vi "MiniProject.vi"() -> ()   [LabVIEW 2021]
panel:
  out "LDR Estimated Lux":dbl
  out "Calculated (V)":dbl
  out "Too Dim 2":bool
  out "Too Bright 2":bool
  out "Raw Voltage (V)":dbl
  out "Average Measured (V)":dbl
  out "Too Dim":bool
  out "Too Bright":bool
  in  "Offset (%)":dbl min=0.0 max=1.0 step=0.01
  out "Reading Range":T1(graph)
  out "LDR Measured Resistance (kOhms)":dbl
  out "Conditioned Signal":T1(graph)
  in  "Stop":bool
  out "Highest Measured Value (V)":dbl
  out "Lowest Measured Value (V)":dbl
  # "500 lux (4.55V)"
  # "100 lux (3.33V)"
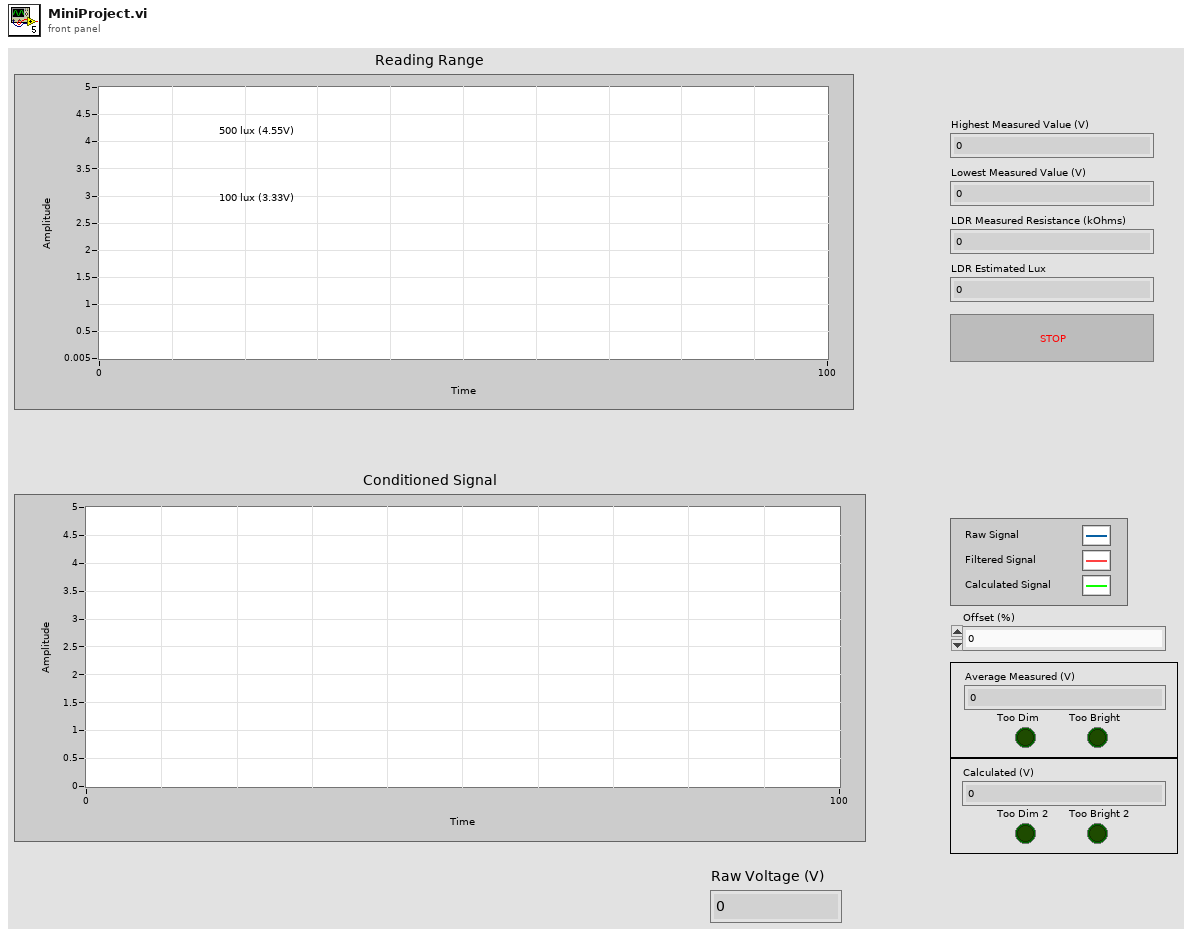
[diagram p1: front panel]
types:
  T1 = cluster{"Voltage Output 1":dbl, "Voltage Output 2":dbl, "Calculated":dbl}
  T2 = enum16{"open", "replace", "create", "open or create", "replace or create", "replace or create with confirmation"}
  T3 = cluster{"Voltage Output 2":dbl, "Min Value":dbl, "Max Value":dbl}
  T4 = cluster{"Voltage Output 2":dbl, dbl, "Calculated":dbl}
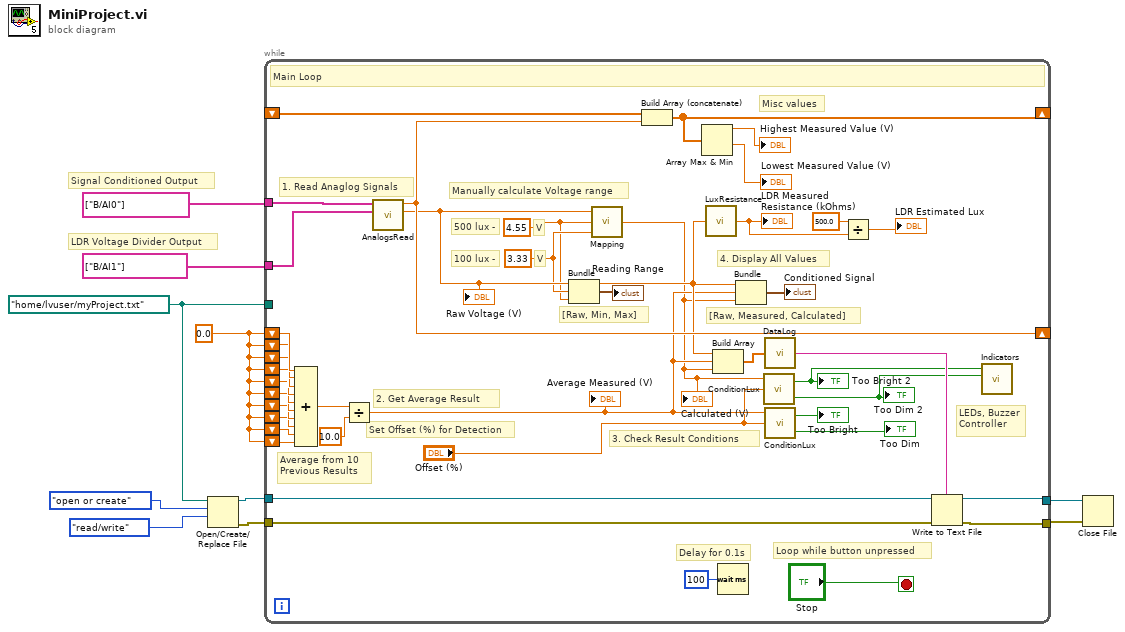
[diagram p0: block diagram]
diagram:
  w5 = path "/home/lvuser/myProject.txt" ("Logfile Location Path")
  w8 = 0.0 ("Voltage Output 2")
  # "LDR Voltage Divider Output"
  # "Signal Conditioned Output"
  n1 = Open/Create/Replace File(file path (use dialog)=w5, operation (0:open)=T2."open or create", access (0:read/write)=enum16{"read/write", "read-only", "write-only"}."read/write") -> (refnum out=w2:refnum<file>, error out=w1:errorcluster)  [unwired: 3 in, 1 out]
  n2 = while {
    tunnel: tag[] ["B/AI0"] ("Analog Input 1") -> [w34]
    tunnel: tag[] ["B/AI1"] ("Analog Input 2") -> [w33]
    shift-right: [w32] -> _
    shift-left: w8 -> [w52]
    shift-left: w8 -> [w51]
    shift-left: w8 -> [w50]
    shift-left: w8 -> [w49]
    shift-left: w8 -> [w48]
    shift-left: w8 -> [w47]
    shift-left: w8 -> [w46]
    shift-left: w8 -> [w45]
    shift-left: w8 -> [w44]
    shift-left: w8 -> [w43]
    shift-right: [w37] -> _
    shift-left: _ -> [w38]
    tunnel: w5 -> [_]
    tunnel: [w17] -> w7
    tunnel: [w16] -> w6
    tunnel: w2 -> [w14]
    tunnel: w1 -> [w13]
    stop <- "Stop" stop-if-true
    w28 = 3.33 ("Min Value")
    w27 = 4.55 ("Max Value")
    # "LEDs, Buzzer\nController"
    # "Set Offset (%) for Detection"
    # "4. Display All Values"
    # "3. Check Result Conditions"
    # "Delay for 0.1s"
    # "2. Get Average Result"
    # "Loop while button unpressed"
    # "V"
    # "V"
    # "1. Read Anaglog Signals"
    # "Misc values"
    # "[Raw, Measured, Calculated]"
    # "[Raw, Min, Max]"
    # "100 lux -"
    # "500 lux -"
    # "Manually calculate Voltage range"
    # "Average from 10 \nPrevious Results"
    # "Main Loop"
    n3 = Compound Arithmetic op=ADD(w52, w51, w50, w49, w48, w47, w46, w45, w44, w43) -> (w42:dbl)
    n4 = Divide(x=w42, y=10.0) -> (x/y=w26:dbl)
    "Average Measured (V)" <- w26
    n5 = call "AnalogsRead.vi"("Analog Input 2"=w33, "Analog Input 1"=w34) -> ("Voltage Output 2"=w30:dbl, "Voltage Output 1"=w32:dbl)  [unwired: 7 in, 1 out]
    "Raw Voltage (V)" <- w30
    n6 = Bundle("Voltage Output 2"=w30, "Min Value"=w28, "Max Value"=w27) -> (→"Reading Range":T3)  [unwired: 1 in]
    n7 = call "Mapping.vi"("Min Value"=w28, "Max Value"=w27, "Raw Signal"=w30) -> ("Calculated"=w22:dbl)
    "Calculated (V)" <- w22
    n8 = Build Array (concatenate)(w38, w32) -> (w37:dbl[])
    n9 = Array Max & Min(array=w37) -> (max value=→"Highest Measured Value (V)":dbl, min value=→"Lowest Measured Value (V)":dbl)  [unwired: 2 out]
    n10 = call "LuxResistance.vi"("Vout"=w30) -> ("Resistance (kOhms)"=w21:dbl)
    "LDR Measured Resistance (kOhms)" <- w21
    n11 = Build Array(w30, w26, w22) -> (w18:dbl[])
    n12 = Wait (ms)(milliseconds to wait=u32 100) -> ()  [unwired: 1 out]
    n13 = Bundle("Voltage Output 2"=w30, w26, "Calculated"=w22) -> (→"Conditioned Signal":T4)  [unwired: 1 in]
    n14 = call "ConditionLux.vi"("Offset"="Offset (%)", "Input"=w22) -> ("Underlimit"=w12:bool, "Overlimit"=w11:bool)  [unwired: 1 in]
    "Too Bright 2" <- w11
    "Too Dim 2" <- w12
    n15 = call "DataLog.vi"("array"=w18) -> ("Result"=w15:string)
    n16 = call "ConditionLux.vi"("Offset"="Offset (%)", "Input"=w26) -> ("Underlimit"=→"Too Dim":bool, "Overlimit"=→"Too Bright":bool)  [unwired: 1 in]
    n17 = Divide(x=500.0, y=w21) -> (x/y=→"LDR Estimated Lux":dbl)
    n18 = Write to Text File(file (use dialog)=w14, text=w15, error in=w13) -> (refnum out=w17:refnum<file>, error out=w16:errorcluster)  [unwired: 1 in, 1 out]
    n19 = call "Indicators.vi"("Overlimit Value"=w11, "Underlimit Value"=w12) -> ()  [unwired: 4 in]
  }
  n20 = Close File(refnum=w7, error in=w6) -> ()  [unwired: 2 out]
